vi "Buffer_Index.vi"(7 "Mode":enum16{"Clear", "Add", "Del", "Output"}(ring), 8 "Delete Position(row)":i32, 10 "End Index":i32, 11 "Start Index":i32) -> (3 "Output Index":i32[][](array[numeric]))   [LabVIEW 2015]
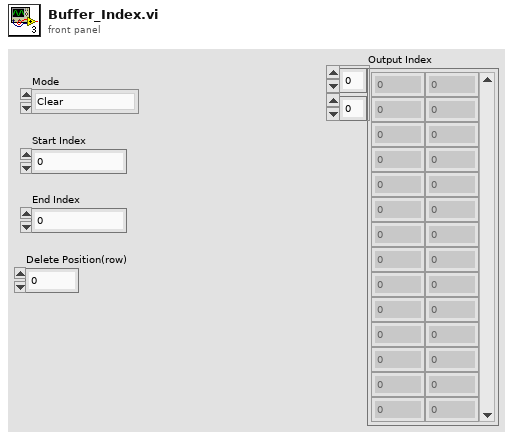
[diagram p1: front panel]
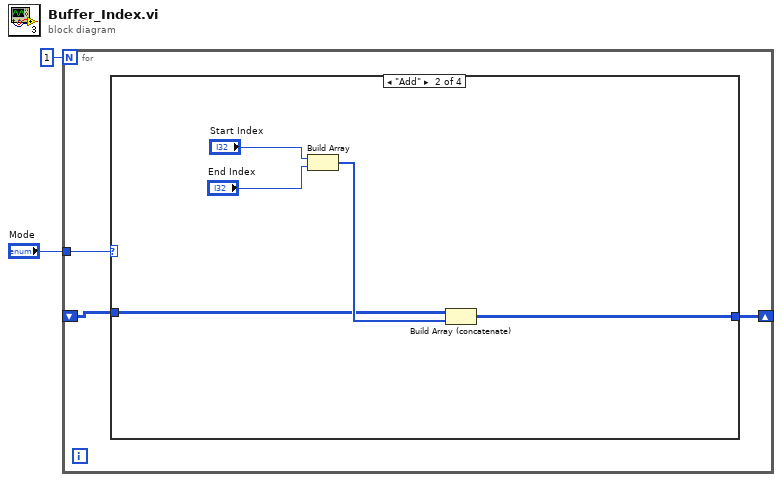
[diagram p0: block diagram]
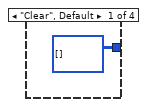
[diagram p2: hidden frame]
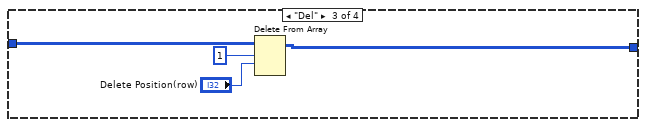
[diagram p3: hidden frame]
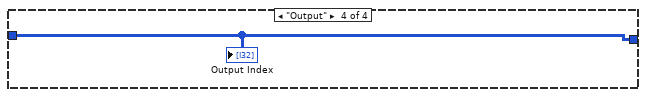
[diagram p4: hidden frame]
diagram:
  n1 = for {
    N: 1 -> [_]
    tunnel: "Mode" -> [w5]
    shift-right: [w4] -> _
    shift-left: _ -> [w3]
    n2 = case shown="\"Add\"" w5 {
      tunnel: [i32[][] [] w8 w12 w16] -> w4
      tunnel: w3 -> [_ w7 w15 w16]
      frame "Clear", Default {
      }
      frame "Add" {
        n3 = Build Array("Start Index", "End Index") -> (w9:i32[])
        n4 = Build Array (concatenate)(w7, w9) -> (w8:i32[][])
      }
      frame "Del" {
        n5 = Delete From Array(array=w15, length=1 ("길이"), index (row)="Delete Position(row)") -> (array with subset deleted=w12:i32[][])  [unwired: 1 in, 1 out]
      }
      frame "Output" {
        "Output Index" <- w16
      }
    }
  }
